vi "ProcessGlobals.vi"(0 "String":string, 1 "String 2":string) -> ()   [LabVIEW 2017]
uses:
  GlobalVars.vi
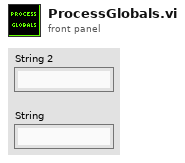
[diagram p1: front panel]
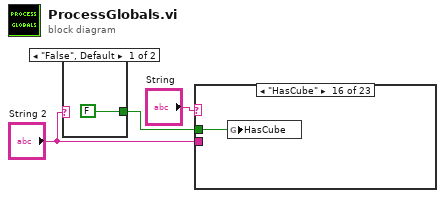
[diagram p0: block diagram]
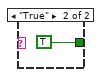
[diagram p2: hidden frame]
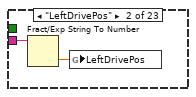
[diagram p4: hidden frame]
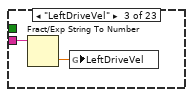
[diagram p5: hidden frame]
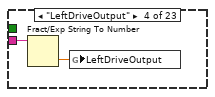
[diagram p6: hidden frame]
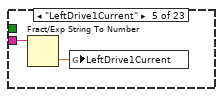
[diagram p7: hidden frame]
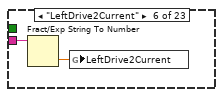
[diagram p8: hidden frame]
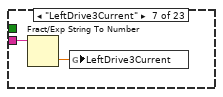
[diagram p9: hidden frame]
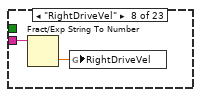
[diagram p10: hidden frame]
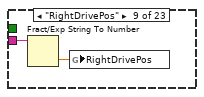
[diagram p11: hidden frame]
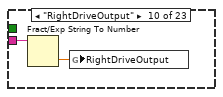
[diagram p12: hidden frame]
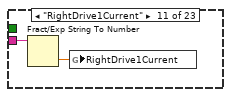
[diagram p13: hidden frame]
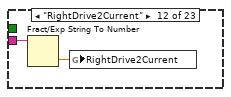
[diagram p14: hidden frame]
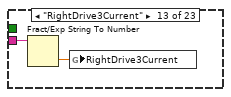
[diagram p15: hidden frame]
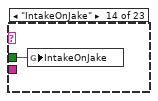
[diagram p16: hidden frame]
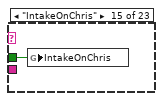
[diagram p17: hidden frame]
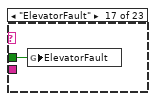
[diagram p18: hidden frame]
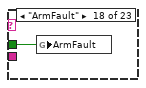
[diagram p19: hidden frame]
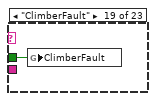
[diagram p20: hidden frame]
diagram:
  n1 = case shown="\"False\", Default" "String 2" {
    tunnel: [FALSE TRUE] -> w2
    frame "False", Default {
    }
    frame "True" {
    }
  }
  n2 = case shown="\"HasCube\"" "String" {
    tunnel: w2 -> [_ _ _ _ _ _ _ _ _ _ _ _ _ w30 w31 w32 w33 w34 w35 _ _ _ _]
    tunnel: "String 2" -> [_ w6 w8 w10 w12 w14 w16 w18 w20 w22 w24 w26 w28 _ _ _ _ _ _ w36 w38 w40 w42]
    frame "False", Default {
    }
    frame "LeftDrivePos" {
      n3 = Fract/Exp String To Number(string=w6) -> (number=w7:dbl)  [unwired: 3 in, 1 out]
      n4 = global write "GlobalVars.vi" "LeftDrivePos"(w7) -> ()
    }
    frame "LeftDriveVel" {
      n5 = Fract/Exp String To Number(string=w8) -> (number=w9:dbl)  [unwired: 3 in, 1 out]
      n6 = global write "GlobalVars.vi" "LeftDriveVel"(w9) -> ()
    }
    frame "LeftDriveOutput" {
      n7 = Fract/Exp String To Number(string=w10) -> (number=w11:dbl)  [unwired: 3 in, 1 out]
      n8 = global write "GlobalVars.vi" "LeftDriveOutput"(w11) -> ()
    }
    frame "LeftDrive1Current" {
      n9 = Fract/Exp String To Number(string=w12) -> (number=w13:dbl)  [unwired: 3 in, 1 out]
      n10 = global write "GlobalVars.vi" "LeftDrive1Current"(w13) -> ()
    }
    frame "LeftDrive2Current" {
      n11 = Fract/Exp String To Number(string=w14) -> (number=w15:dbl)  [unwired: 3 in, 1 out]
      n12 = global write "GlobalVars.vi" "LeftDrive2Current"(w15) -> ()
    }
    frame "LeftDrive3Current" {
      n13 = Fract/Exp String To Number(string=w16) -> (number=w17:dbl)  [unwired: 3 in, 1 out]
      n14 = global write "GlobalVars.vi" "LeftDrive3Current"(w17) -> ()
    }
    frame "RightDriveVel" {
      n15 = Fract/Exp String To Number(string=w18) -> (number=w19:dbl)  [unwired: 3 in, 1 out]
      n16 = global write "GlobalVars.vi" "RightDriveVel"(w19) -> ()
    }
    frame "RightDrivePos" {
      n17 = Fract/Exp String To Number(string=w20) -> (number=w21:dbl)  [unwired: 3 in, 1 out]
      n18 = global write "GlobalVars.vi" "RightDrivePos"(w21) -> ()
    }
    frame "RightDriveOutput" {
      n19 = Fract/Exp String To Number(string=w22) -> (number=w23:dbl)  [unwired: 3 in, 1 out]
      n20 = global write "GlobalVars.vi" "RightDriveOutput"(w23) -> ()
    }
    frame "RightDrive1Current" {
      n21 = Fract/Exp String To Number(string=w24) -> (number=w25:dbl)  [unwired: 3 in, 1 out]
      n22 = global write "GlobalVars.vi" "RightDrive1Current"(w25) -> ()
    }
    frame "RightDrive2Current" {
      n23 = Fract/Exp String To Number(string=w26) -> (number=w27:dbl)  [unwired: 3 in, 1 out]
      n24 = global write "GlobalVars.vi" "RightDrive2Current"(w27) -> ()
    }
    frame "RightDrive3Current" {
      n25 = Fract/Exp String To Number(string=w28) -> (number=w29:dbl)  [unwired: 3 in, 1 out]
      n26 = global write "GlobalVars.vi" "RightDrive3Current"(w29) -> ()
    }
    frame "IntakeOnJake" {
      n27 = global write "GlobalVars.vi" "IntakeOnJake"(w30) -> ()
    }
    frame "IntakeOnChris" {
      n28 = global write "GlobalVars.vi" "IntakeOnChris"(w31) -> ()
    }
    frame "HasCube" {
      n29 = global write "GlobalVars.vi" "HasCube"(w32) -> ()
    }
    frame "ElevatorFault" {
      n30 = global write "GlobalVars.vi" "ElevatorFault"(w33) -> ()
    }
    frame "ArmFault" {
      n31 = global write "GlobalVars.vi" "ArmFault"(w34) -> ()
    }
    frame "ClimberFault" {
      n32 = global write "GlobalVars.vi" "ClimberFault"(w35) -> ()
    }
    frame "ElevatorPositionAct" {
      n33 = Fract/Exp String To Number(string=w36) -> (number=w37:dbl)  [unwired: 3 in, 1 out]
      n34 = global write "GlobalVars.vi" "ElevatorPositionAct"(w37) -> ()
    }
    frame "ElevatorPosReq" {
      n35 = Fract/Exp String To Number(string=w38) -> (number=w39:dbl)  [unwired: 3 in, 1 out]
      n36 = global write "GlobalVars.vi" "ElevatorPositionReq"(w39) -> ()
    }
    frame "ArmAngle" {
      n37 = Fract/Exp String To Number(string=w40) -> (number=w41:dbl)  [unwired: 3 in, 1 out]
      n38 = global write "GlobalVars.vi" "ArmAngle"(w41) -> ()
    }
    frame "ArmLength" {
      n39 = Fract/Exp String To Number(string=w42) -> (number=w43:dbl)  [unwired: 3 in, 1 out]
      n40 = global write "GlobalVars.vi" "ArmLength"(w43) -> ()
    }
  }
